vi "OszilloskopManuellVI.vi"(0 "Maximaler absoluter Wert":dbl=5.0 format="%0.2f", 1 "Speichern":bool, 2 "physical channels":tag="Dev1/ai0", 3 "Anzahl der Messpunkte":i32=4000, 4 "stopp":bool, 5 "Rate":dbl=40000.0 format="%0.2f") -> (6 "Zeitbild":waveform(dbl)(graph), 7 "Spektralanalyse":cluster{"f0":dbl, "df":dbl, "magnitude":dbl[]}(graph), 8 "Spektralanalyse Hanning":cluster{"f0":dbl, "df":dbl, "magnitude":dbl[]}(graph))   [LabVIEW 2017]
uses:
  <vilib>/Utility/error.llb/DialogType.ctl
  <vilib>/DAQmx/read.llb/DAQmx Read (Analog Wfm 1Chan NSamp).vi
  <vilib>/DAQmx/create/channels.llb/DAQmx Create Channel (AI-Voltage-Basic).vi
  <vilib>/DAQmx/configure/timing.llb/DAQmx Timing (Sample Clock).vi
  <vilib>/DAQmx/miscellaneous.llb/DAQmx Fill In Error Info.vi
  <vilib>/express/express analysis/Spectral/Block/exnSpectralBlock spectral measurements power poly.vi
  <vilib>/express/express analysis/Spectral/Block/exnSpectralBlock spectral measurements power WFM.vi
  <vilib>/Utility/file.llb/Write Delimited Spreadsheet (DBL).vi
  <vilib>/express/express analysis/Spectral/XNode/ExpressSpectralMeasurementsBlockNode.xnode
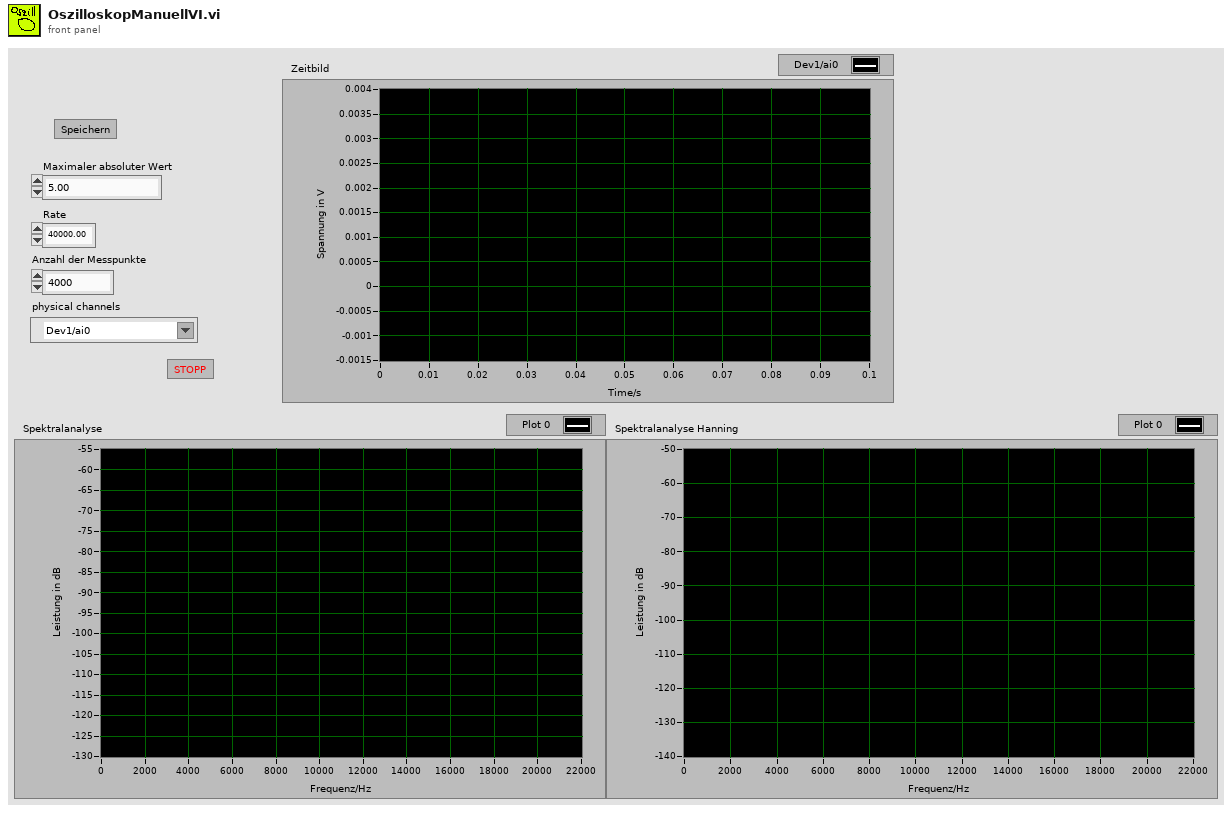
[diagram p1: front panel]
types:
  T1 = cluster{"averaging mode":u16, "weighting mode":u16, "number of averages":u32}
  T2 = cluster{"dB On (F)":bool, "unwrap phase (F)":bool, "convert to degree (F)":bool}
  T3 = typedef "DialogType.ctl" = u16
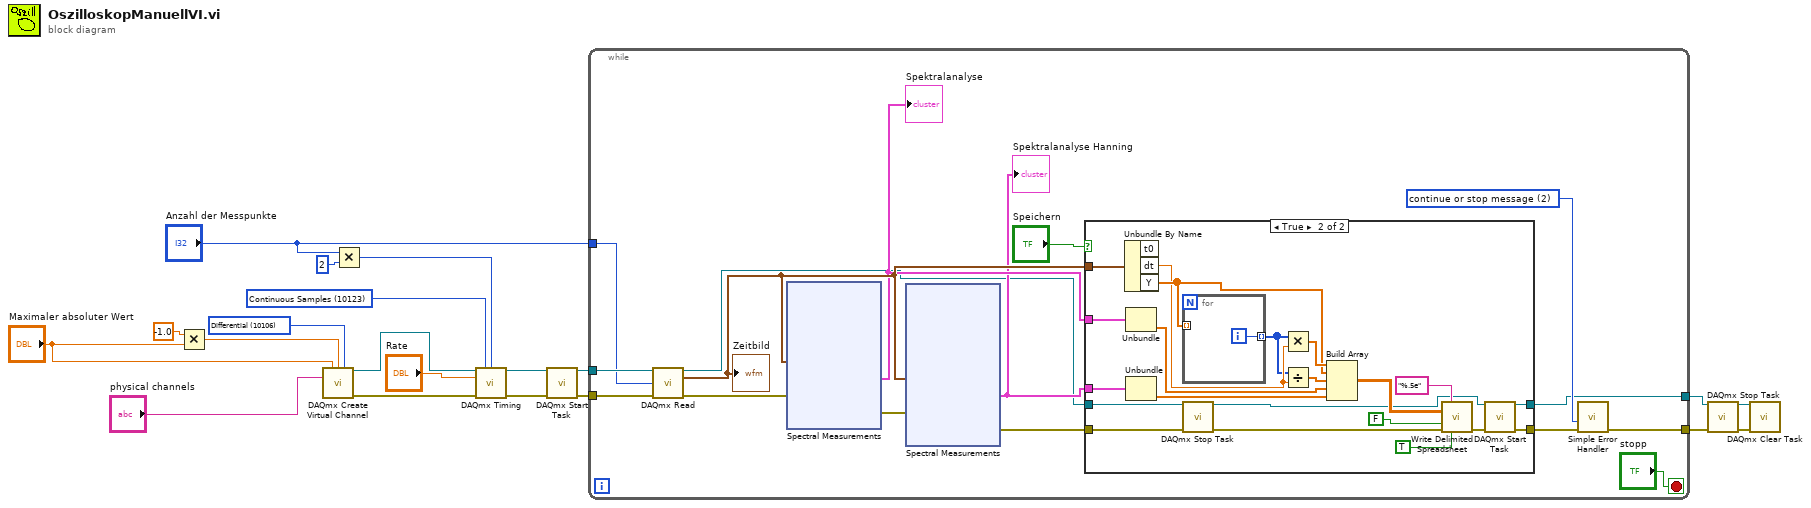
[diagram p0: block diagram]
diagram:
  w14 = 10106 items=["Default"=-1, "RSE"=10083, "NRSE"=10078, "Differential"=10106, "Pseudodifferential"=12529] ("input terminal configuration")
  w15 = 10123 items=["Finite Samples"=10178, "Continuous Samples"=10123, "Hardware Timed Single Point"=12522] ("sample mode")
  n1 = Multiply(x=-1.0, y="Maximaler absoluter Wert") -> (x*y=w13:dbl)
  n2 = call-poly <vilib>:"DAQmx Create Virtual Channel.vi"("maximum value"="Maximaler absoluter Wert", "minimum value"=w13, "input terminal configuration"=w14, "physical channels"="physical channels") -> ("task out"=w19:refnum<k21>, "error out"=w20:errorcluster)  [unwired: 10 in]
  n3 = Multiply(x="Anzahl der Messpunkte", y=2) -> (x*y=w2:i32)
  n4 = call-poly <vilib>:"DAQmx Timing.vi"("task/channels in"=w19, "sample mode"=w15, "samples per channel"=w2, "rate"="Rate", "error in"=w20) -> ("task out"=w17:refnum<k21>, "error out"=w16:errorcluster)  [unwired: 9 in]
  n5 = call <vilib>:"DAQmx Start Task.vi"("task/channels in"=w17, "error in"=w16) -> ("task out"=w8:refnum<k21>, "error out"=w9:errorcluster)  [unwired: 12 in]
  n6 = while {
    tunnel: w9 -> [w34]
    tunnel: w8 -> [w35]
    tunnel: "Anzahl der Messpunkte" -> [w33]
    tunnel: [w32] -> w6
    tunnel: [w21] -> w5
    stop <- "stopp" stop-if-true
    w31 = T3 2 items=["no dialog", "OK message", "continue or stop message", "OK message + warnings", "continue/stop + warnings"] ("type of dialog (OK msg:1)")
    n7 = call-poly <vilib>:"DAQmx Read.vi"("task/channels in"=w35, "number of samples per channel"=w33, "error in"=w34) -> ("task out"=w22:refnum<k21>, "data"=w26:waveform(dbl), "error out"=w30:errorcluster)  [unwired: 10 in]
    "Zeitbild" <- w26
    n8 = xnode "Spectral Measurements"("Signals"=w26, "error in (no error)"=w30) -> ("Power Spectrum"=w25:cluster{"f0":dbl, "df":dbl, "magnitude":dbl[]}, "error out"=w29:errorcluster)
    "Spektralanalyse" <- w25
    n9 = xnode "Spectral Measurements"("Signals"=w26, "error in (no error)"=w29) -> ("Power Spectrum"=w24:cluster{"f0":dbl, "df":dbl, "magnitude":dbl[]}, "error out"=w28:errorcluster)
    "Spektralanalyse Hanning" <- w24
    n10 = case shown="True" "Speichern" {
      tunnel: w28 -> [w38 w45]
      tunnel: [w38 w44] -> w27
      tunnel: w26 -> [_ w46]
      tunnel: w25 -> [_ w56]
      tunnel: w24 -> [_ w55]
      tunnel: w22 -> [w37 w43]
      tunnel: [w37 w41] -> w21
      frame False {
      }
      frame True {
        n11 = Unbundle By Name(w46) -> ("dt"=w49:dbl, "Y"=w50:dbl[])  [unwired: 1 out]
        n12 = Unbundle(w56) -> ("magnitude"=w53:dbl[])  [unwired: 2 out]
        n13 = Unbundle(w55) -> ("magnitude"=w54:dbl[])  [unwired: 2 out]
        n14 = for {
          tunnel: [w60] -> w48 mode=indexing
          tunnel: w50 -> [_] mode=indexing
          i -> [w60]
        }
        n15 = call <vilib>:"DAQmx Stop Task.vi"("task/channels in"=w43, "error in"=w45) -> ("task out"=w42:refnum<k21>, "error out"=w40:errorcluster)  [unwired: 12 in]
        n16 = Multiply(x=w48, y=w49) -> (x*y=w51:dbl[])
        n17 = Divide(x=w48, y=w49) -> (x/y=w47:dbl[])
        n18 = Build Array(w51, w50, w47, w53, w54) -> (w52:dbl[][])
        n19 = call-poly <vilib>:"Write Delimited Spreadsheet.vi"("format (%.3f)"="%.5e", "2D data"=w52, "append to file? (new file:F)"=FALSE, "error in (no error)"=w40, "transpose? (no:F)"=TRUE) -> ("error out"=w39:errorcluster)  [unwired: 9 in, 1 out]
        n20 = call <vilib>:"DAQmx Start Task.vi"("task/channels in"=w42, "error in"=w39) -> ("task out"=w41:refnum<k21>, "error out"=w44:errorcluster)  [unwired: 12 in]
      }
    }
    n21 = call <vilib>:"Simple Error Handler.vi"("type of dialog (OK msg:1)"=w31, "error in (no error)"=w27) -> ("error out"=w32:errorcluster)  [unwired: 3 in, 4 out]
  }
  n22 = call <vilib>:"DAQmx Stop Task.vi"("task/channels in"=w5, "error in"=w6) -> ("task out"=w7:refnum<k21>, "error out"=w1:errorcluster)  [unwired: 12 in]
  n23 = call <vilib>:"DAQmx Clear Task.vi"("task in"=w7, "error in"=w1) -> ()  [unwired: 13 in, 1 out]
